vi "GetControlLocation.vi"(6 "error in":errorcluster, 7 "Control in":refnum<vi>) -> (0 "error out":errorcluster, 4 "Position":T1, 5 "Bounds":T2)   [LabVIEW 2014, in "Raspberry Pi Compatible Compiler for LabVIEW.lvlib" / "Control.lvclass"]
uses:
  Control.lvclass
  <vilib>/Utility/miscctls.llb/LVBoundsTypeDef.ctl
  <vilib>/Utility/miscctls.llb/LVPositionTypeDef.ctl
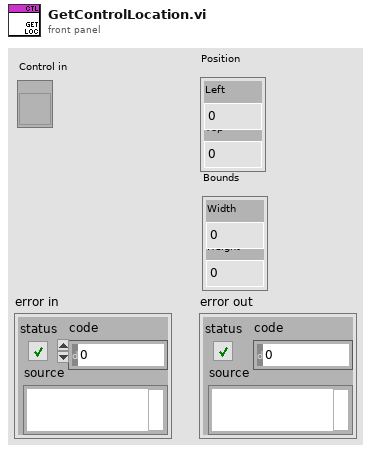
[diagram p1: front panel]
types:
  T1 = typedef "LVPositionTypeDef.ctl" = cluster{"Left":i32, "Top":i32}
  T2 = typedef "LVBoundsTypeDef.ctl" = cluster{"Width":u32, "Height":u32}
  T3 = typedef "LVRectTypeDef.ctl" = cluster{"Left":i16, "Top":i16, "Right":i16, "Bottom":i16}
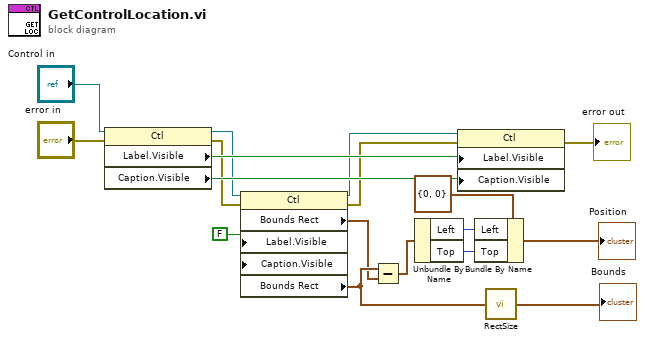
[diagram p0: block diagram]
diagram:
  w5 = FALSE ("Label.Visible")
  n1 = property class="Ctl"(reference="Control in", error in="error in") -> (reference out=w4:refnum<vi>, error out=w3:errorcluster, "Label.Visible"=w16:bool, "Caption.Visible"=w17:bool)
  n2 = property class="Ctl"(reference=w4, error in=w3, "Label.Visible"=w5, "Caption.Visible"=w5) -> (reference out=w15:refnum<vi>, error out=w14:errorcluster, "Bounds Rect"=w6:T3, "Bounds Rect"=w13:T3)
  n3 = Subtract(x=w13, y=w6) -> (x-y=w7:T3)
  n4 = Unbundle By Name(w7) -> ("Left"=w9:i16, "Top"=w10:i16)
  n5 = property class="Ctl"(reference=w15, error in=w14, "Label.Visible"=w16, "Caption.Visible"=w17) -> (error out=→"error out":errorcluster)  [unwired: 1 out]
  n6 = Bundle By Name(cluster=T1 {"Left"=0, "Top"=0} ("Position"), "Left"=w9, "Top"=w10) -> (→"Position":T1)
  n7 = call <vilib>:"RectSize.vi"("rect"=w13) -> ("point"=→"Bounds":cluster{"x":i16, "y":i16})
